vi "CPP-BLplotter.vi"(0 "Plot Array":cluster{dbl[], dbl[]}[](array[cluster])=[{[500.0, 500.0, 953.54, 215.0, 270.0, 320.0, 445.0, 525.0, 600.0, 675.0, 750.0, 825.0, 900.0, 960.0, 1010.0, 1060.0], [4.614524, 4.54365, 5.818368, 0.1374656, 0.6662545, 1.465458, 3.619824, 4.848976, 5.887329, 5.940571, 6.152151, 5.717487, 5.600293, 5.40069, 5.154843, 5.121789]}, {[100.0, 150.0, 215.0, 270.0, 320.0, 445.0, 525.0, 600.0, 675.0, 750.0, 825.0, 900.0, 960.0, 1010.0, 1060.0], [0.002314715, -0.00693192, 0.120417, 0.6880509, 1.519176, 3.513709, 5.065183, 6.116033, 6.096773, 5.938465, 5.593788, 5.5597, 5.387002, 5.304077, 4.887903]}] {"?" format="%.2f"; "?" format="%.2f"}, 1 "Job Directory":path=path "/G4_2_HD/Users/paulhayden/Documents/Projects/Westlakes_resolution") -> (2 "Saved Automatically?":bool, 3 "gnuplotScript":string="set term epslatex\nset output \"Plot.eps\"\nset xlabel '$Distance~(m)$'\nset ylabel '$DF~(s/m^3)\\times10^6$'\nset samples 1000\nset pointsize 1.00\nset title '$B38~Centreline~Glc$' 0, 0\nset size 0.75,0.9\n\n#set key 450, -2.5833\n unset key\nset label 1 '~~~~~~~~~~~Angle~(deg)~=~0' at -100, -2.58\nset label 2 '~~~~~~~~~~~Height~(m)~=~5' at -100, -3.27\n set xrange [0 : 500] \n# set autoscale x \n set yrange [0.10000 : 7]\n# set autoscale y \n\nplot \"B38_Centreline_Glc.dat\" index 0 using 1:2 axes x1y1 title '$File=B38R~DDD.xls$' with points 1 1, \\\n\"B38_Centreline_Glc.dat\" index 1 using 1:2 axes x1y1 title '$File=B38R~DDD~1.xls$' with points 1 3", 4 "Plot data file":path)   [LabVIEW 2013]
uses:
  Results_plotter_Global.vi
panel:
  in  "Tab Control":enum32{"Good Shit", "Boring Shit"}(tab)
  out "lambda-":dbl format="%_2g"
  out "lambda+":dbl format="%_2g"
  out "lambda(h)":dbl format="%.3g"
  in  "HeightJitter%":dbl=0.03 min=0.0 max=20.0 step=1.0
  in  "Spectra Folder::":path
  out "Spectrum":cluster{"all rows":dbl[], "all rows":dbl[]}[](graph)
  in  "Cancel Button":bool
  in  "Print Button":bool
  out "U,L(U)":cluster{dbl[], dbl[]}[](graph)
  out "TI,Sigma":cluster{dbl[], dbl[]}[](graph)
  in  "MaxFitFreq":dbl
  in  "U(h)":dbl
  in  "lambdaSpan(%)":dbl
  in  "integralTweak":dbl=1.0 min=0.8 max=1.2 step=0.01
  in  "Use for:":enum16{"\nU", "\nLambda", "\nTI", "\nSigma"}[](array[ring])=[enum."\nU", enum."\nTI", enum."\nSigma", enum."\nLambda"]
  out "Incoming Titles":string[](array[string])
  in  "Plot Title":u16(ring) items=["Title String Only", "Number of Measurements", "Date::", "Profile::", "Multi Run:Start Time:", "Multi Run:Row:Type", "Multi Run:Row:Number", "Point:Time:", "Time:Stamp:", "Measuring:Instrument:Type", "Comments::", "Run:Messages:", "X_{HF}:(mm):", "Y_{HF}:(mm):", "Z_{HF}:(mm):", "X_{5HP}:(mm):", "Y_{5HP}:(mm):", "Z_{5HP}:(mm):", "Repeat::", "U_{HF}/U_{ref}::", "TI_{HF}:%:", "\\sigma_{HF}/U_{ref}::", "L(U):Est:(m)", "U_{5HP}/U_{ref}::", "U_{HF}/U_{5HP}::", "TI_{U(5HP)}:%:", "Vmag_{5HP}/U_{ref}::", "V_{5HP}/U_{5HP}::", "W_{5HP}/U_{5HP}::", "U_{ref}::", "U_{HF}::", "Tau(HF)::", "uhf^2::", "uhf^3/(uhf^2)^1.5::", "(uhf^4/(uhf^2)^2) -3::", "HW (Uhf):Standard Error:in Mean", "HW (Uhf):Standard Error:in Variance", "HW:Cal:", "Vmag_{5HP}::", "U_{5HP}::", "V_{5HP}::", "W_{5HP}::", "Vmag_SD::", "U_SD::", "V_SD::", "W_SD::", "Tau(5HP1)::(nose)", "Tau(5HP2)::(bottom)", "Tau(5HP3)::(top)", "Tau(5HP4)::(side)", "Tau(5HP5)::(side)", "GoodFraction::", "5HP:Mode:", "5HP:ReturnType:", "Reference:Temperature:Used for Corrections", "Atmos:Pressure:Used for Corrections", "Av Analogue:Sampling:Rate", "No of:Analogue:Samples", "No Of:Measurement:Blocks", "Flow:Measurement:Time", "X:(URef):(mm)", "Y:(URef):(mm)", "Z:(URef):(mm)", "Original:Results:Filename", "Current:Data:Filename", "Current:Data File:1st Folder level", "Current:Data File:2nd Folder level", "Current:Data File:3rd Folder level", "Current:Data File:4th Folder level", "Current:File:Number", "Raw:Data:Filename"]
  in  "Filename Max length":i32=255
  out "Final Title":string="B38 Centreline Glc"
  out "Path":path
  in  "Plot Title Post Block":string
  in  "Plot Title Pre Block":string
  in  "Show Script Editor?":bool
  out "t":string
  in  "OpenLogfile?":bool
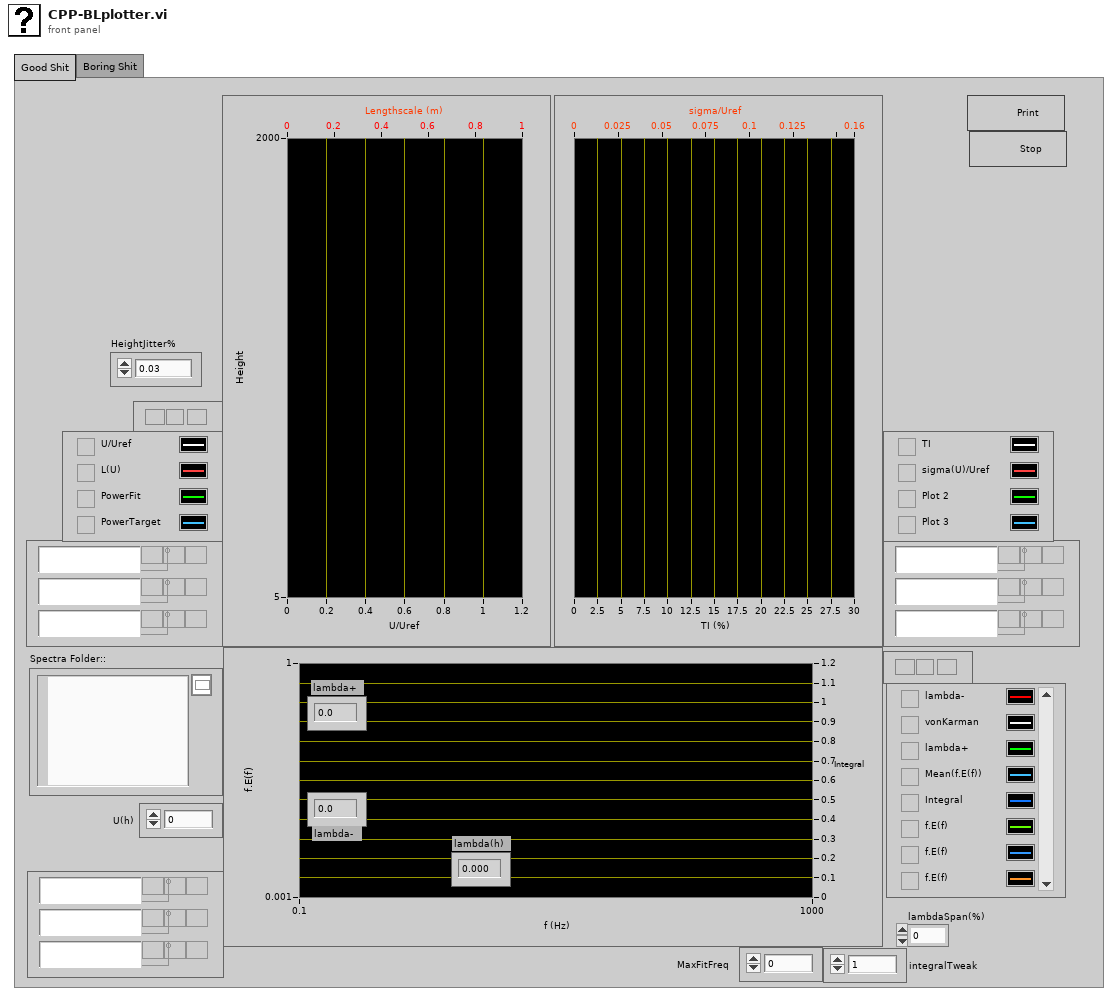
[diagram p1: front panel]
types:
  T1 = typedef "LVRangeTypeDef.ctl" = cluster{"Minimum":dbl, "Maximum":dbl, "Increment":dbl, "Minor Increment":dbl, "Start":dbl}
  T2 = cluster{"Array":dbl[], "best nonlinear fit":dbl[]}
  T3 = typedef "minAndMax.ctl" = cluster{"Min":T4, "Max":T4}
  T4 = typedef "AutoManualNumber.ctl" = cluster{"Auto":bool, "Value":dbl}
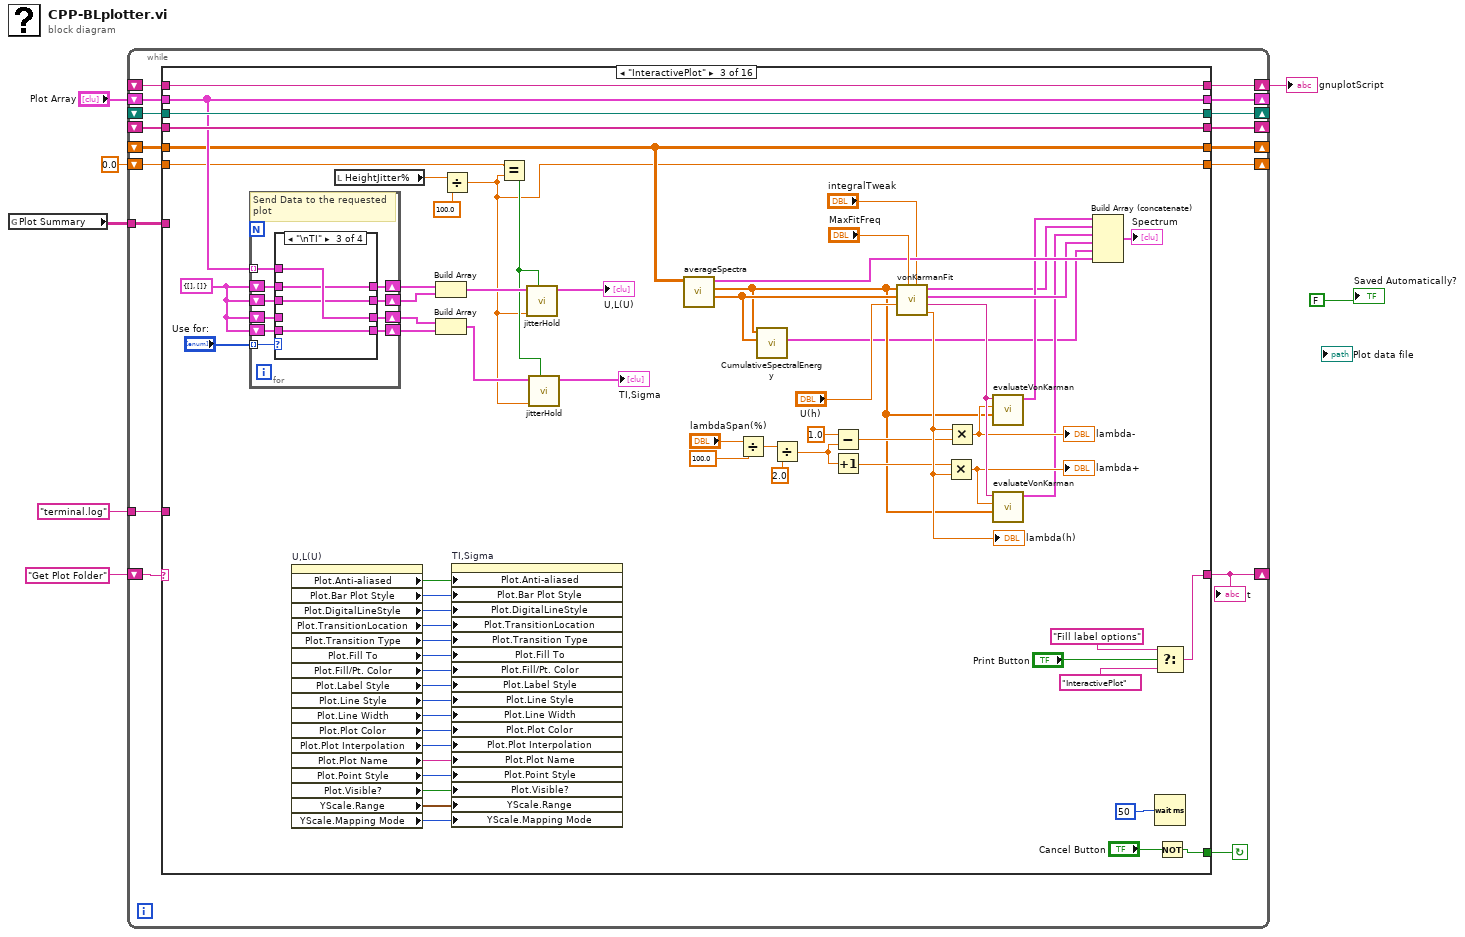
[diagram p0: block diagram]
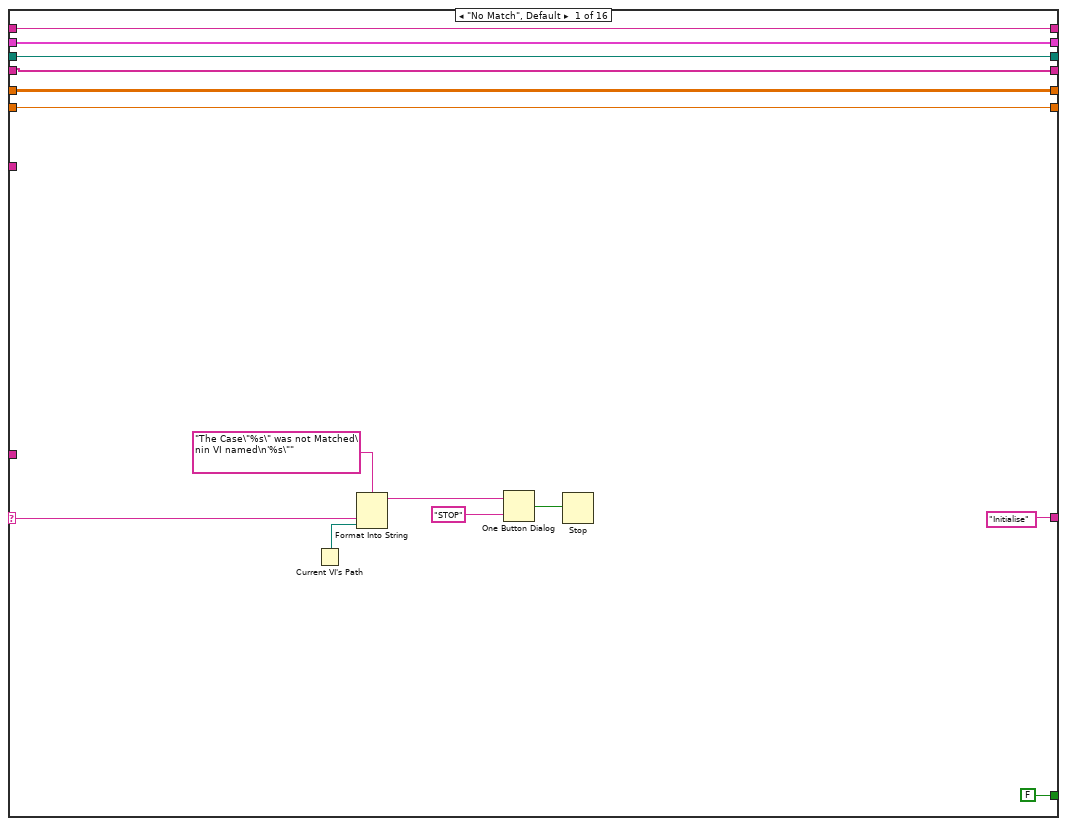
[diagram p2: hidden frame]
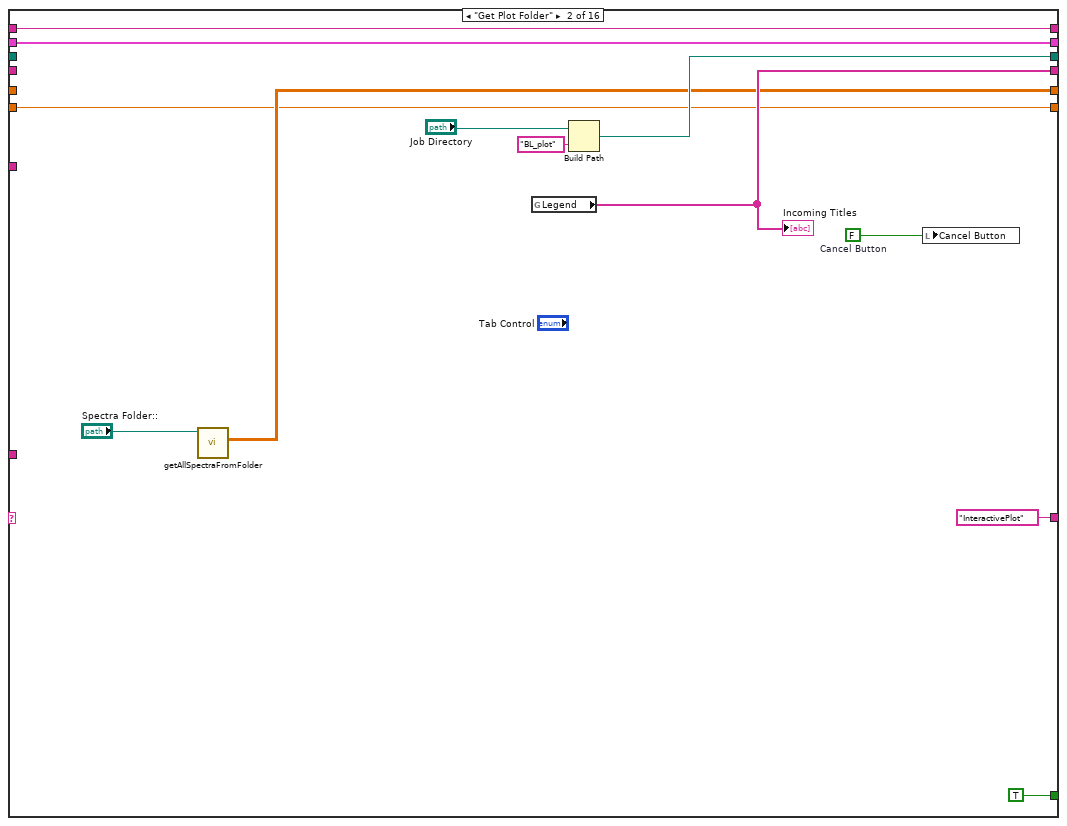
[diagram p3: hidden frame]
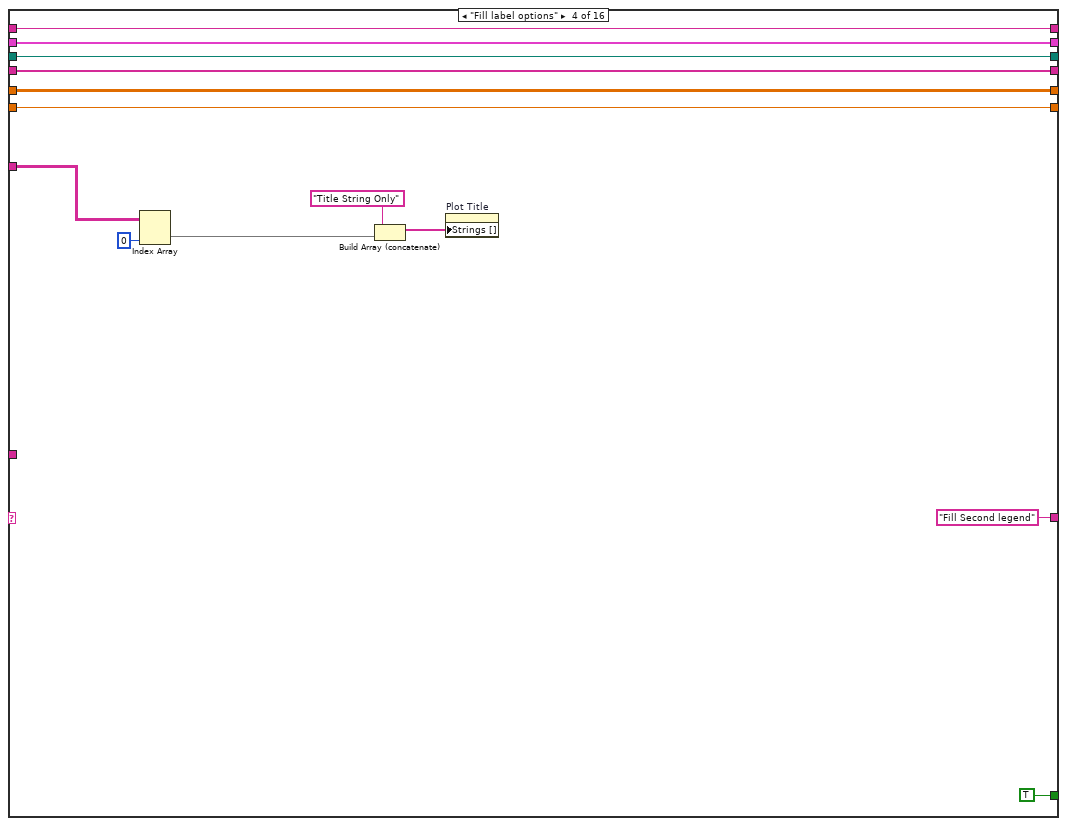
[diagram p7: hidden frame]
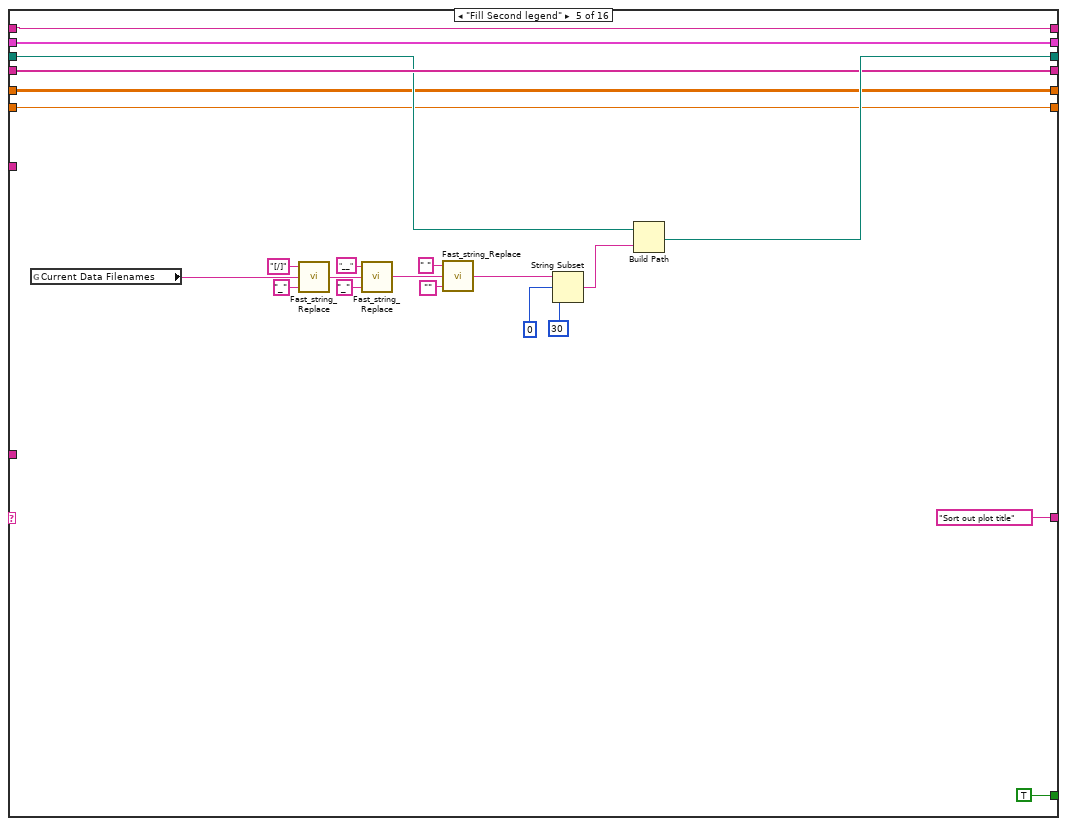
[diagram p8: hidden frame]
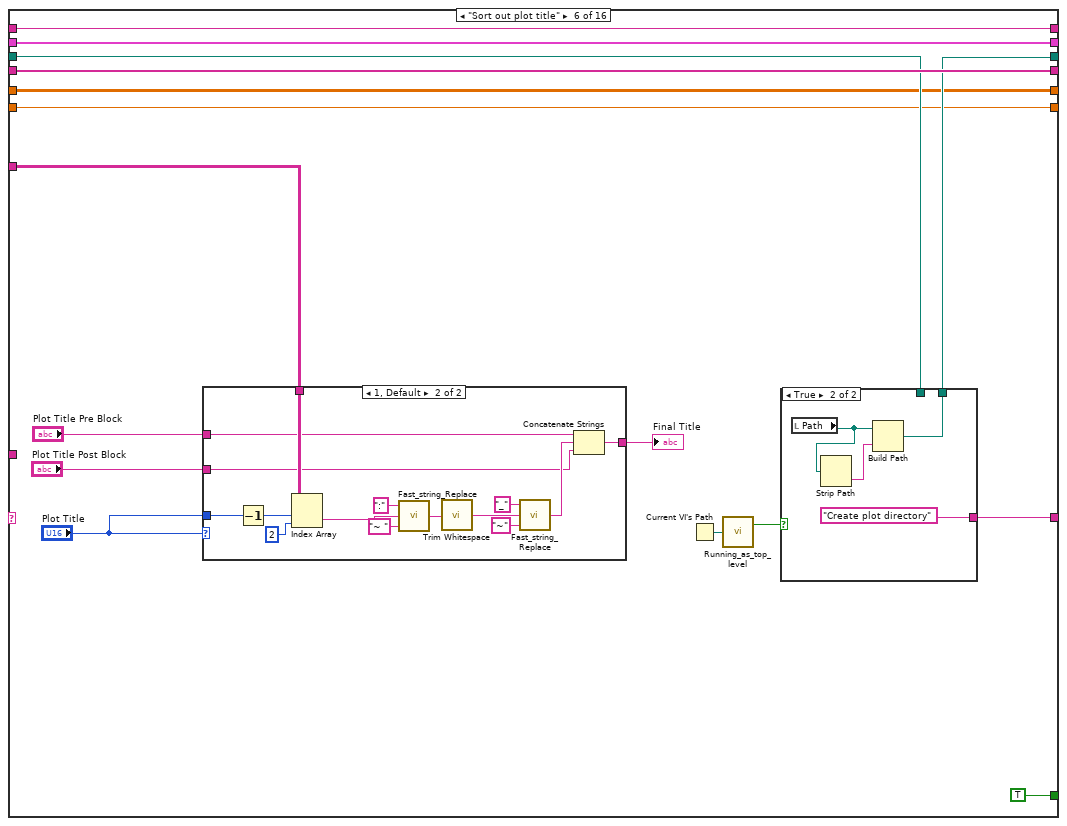
[diagram p9: hidden frame]
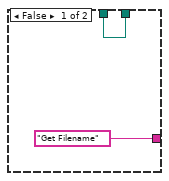
[diagram p10: hidden frame]
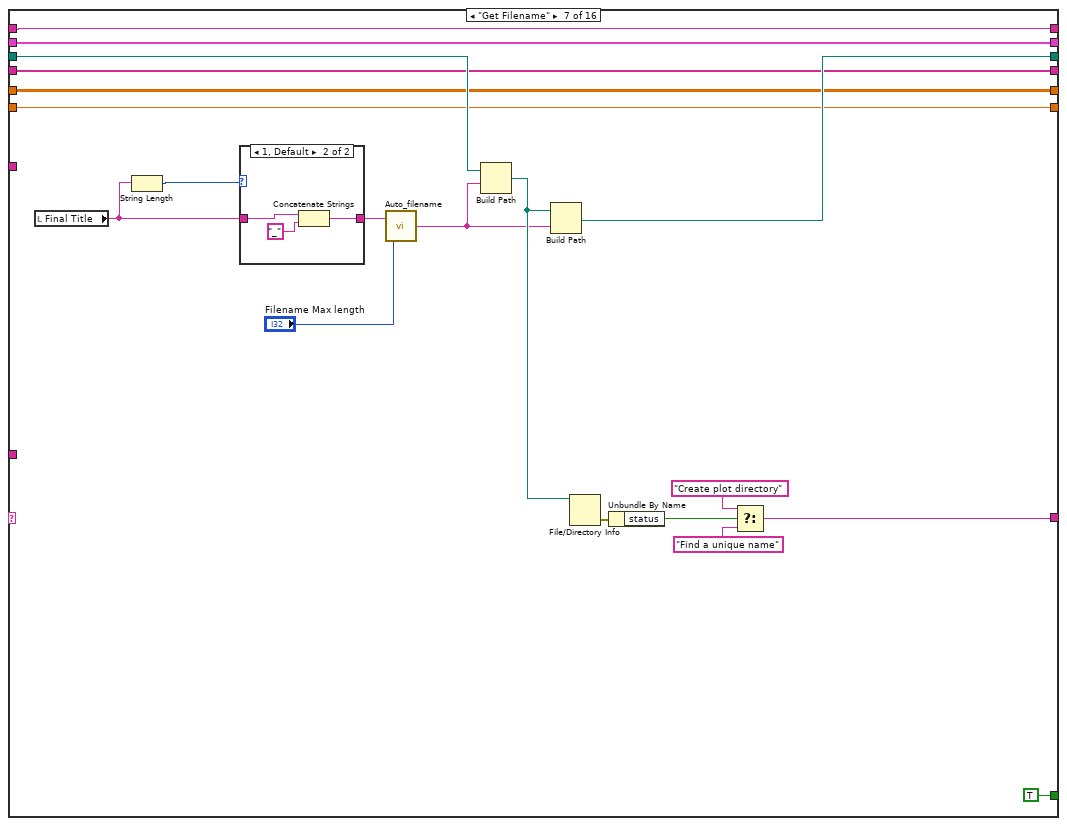
[diagram p12: hidden frame]
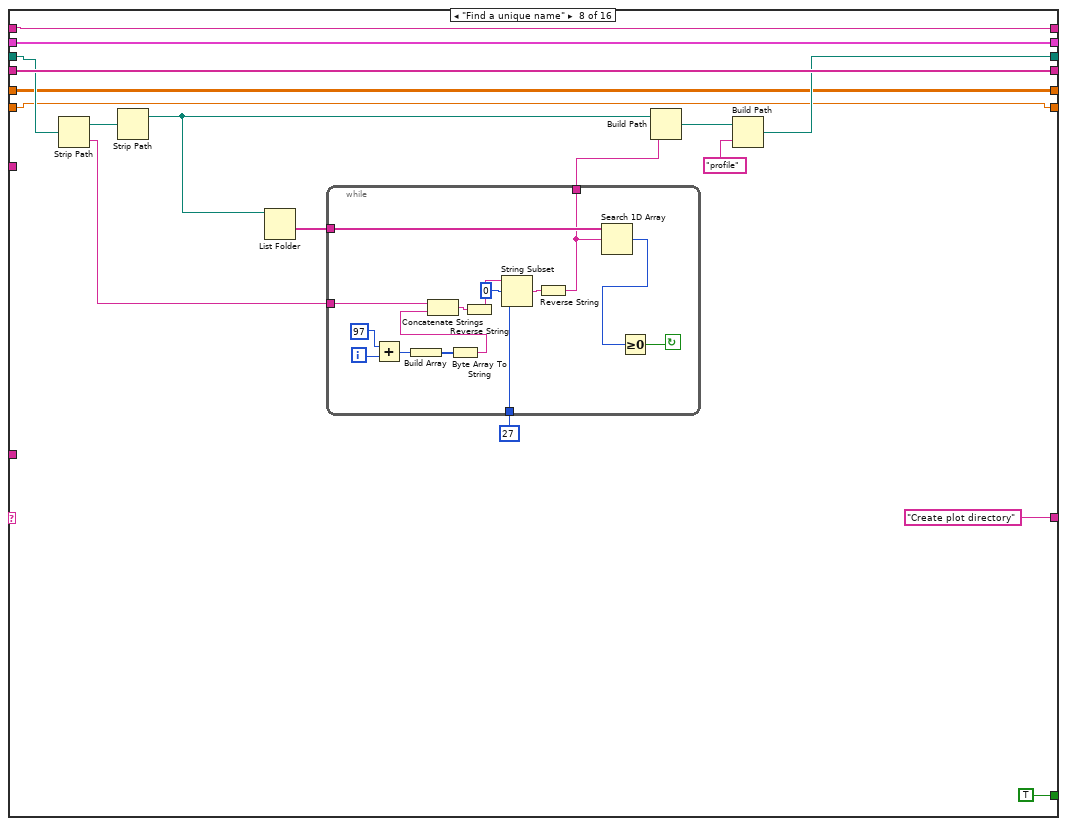
[diagram p14: hidden frame]
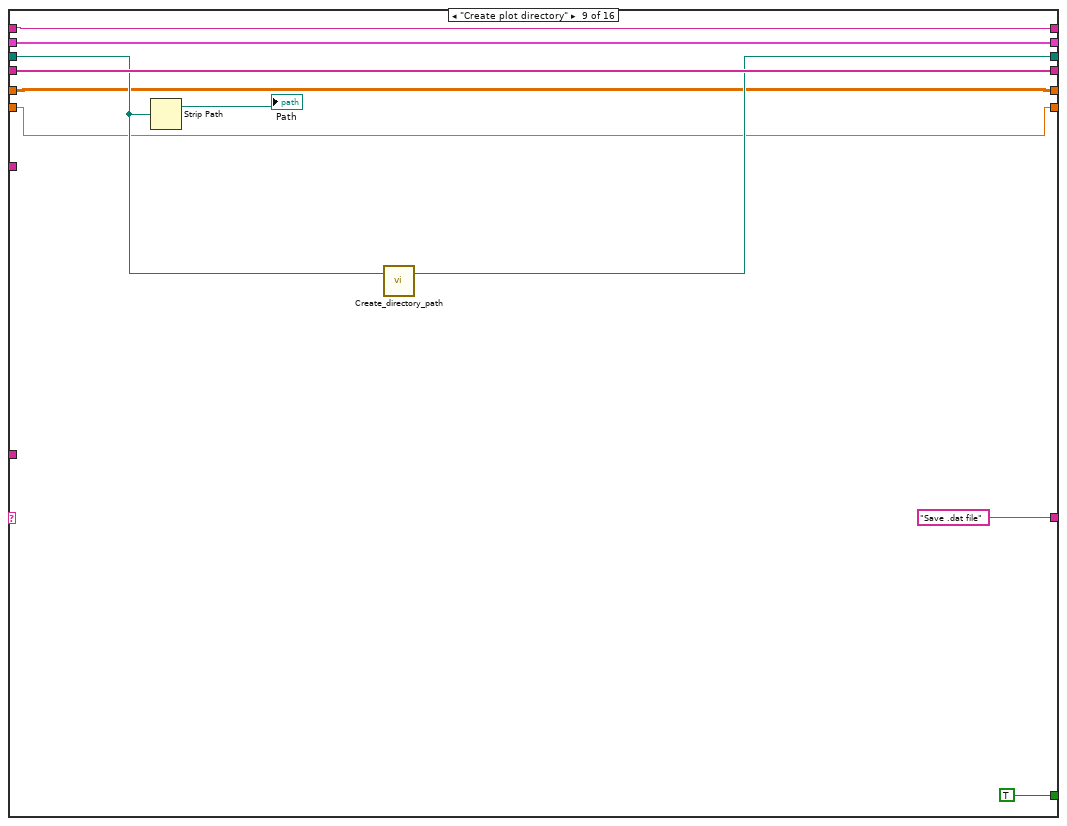
[diagram p15: hidden frame]
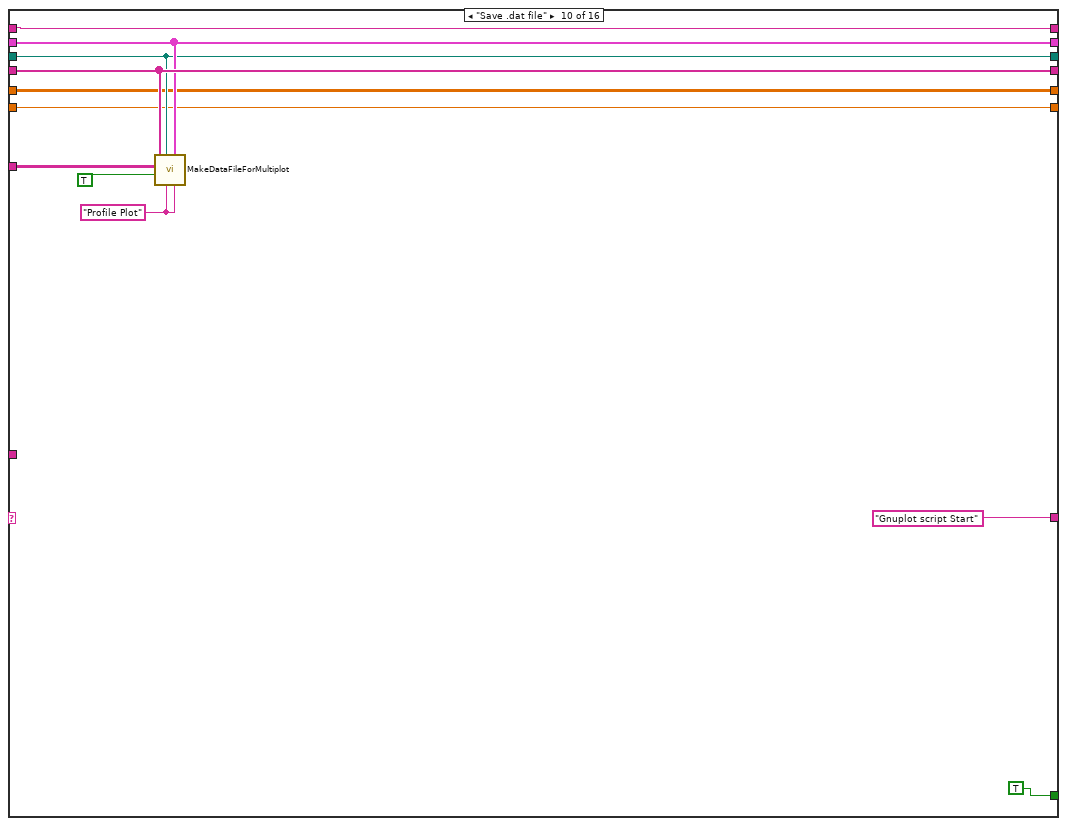
[diagram p16: hidden frame]
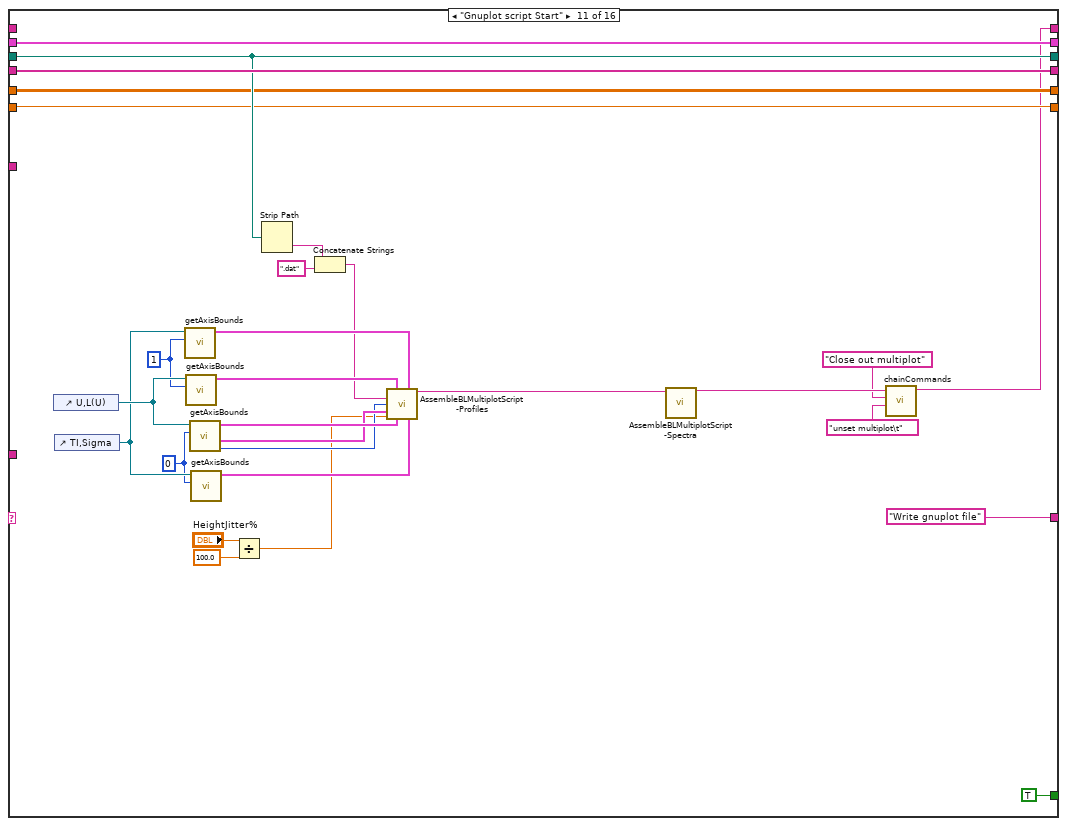
[diagram p17: hidden frame]
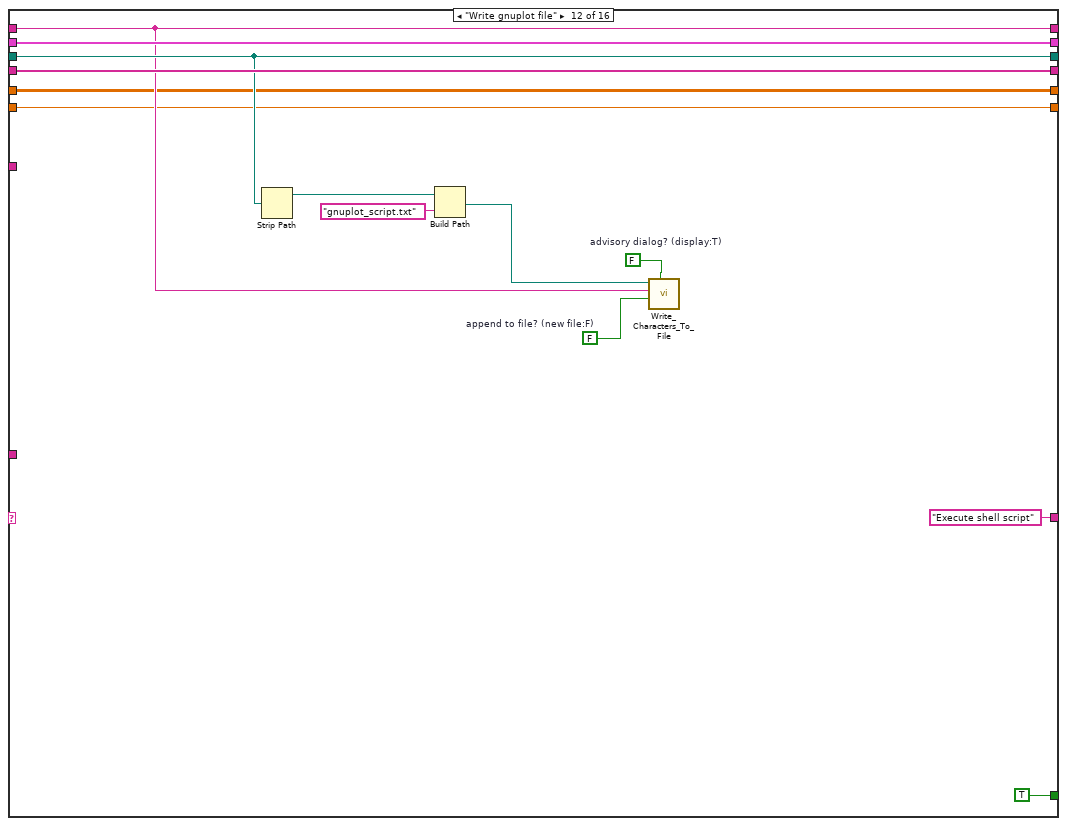
[diagram p18: hidden frame]
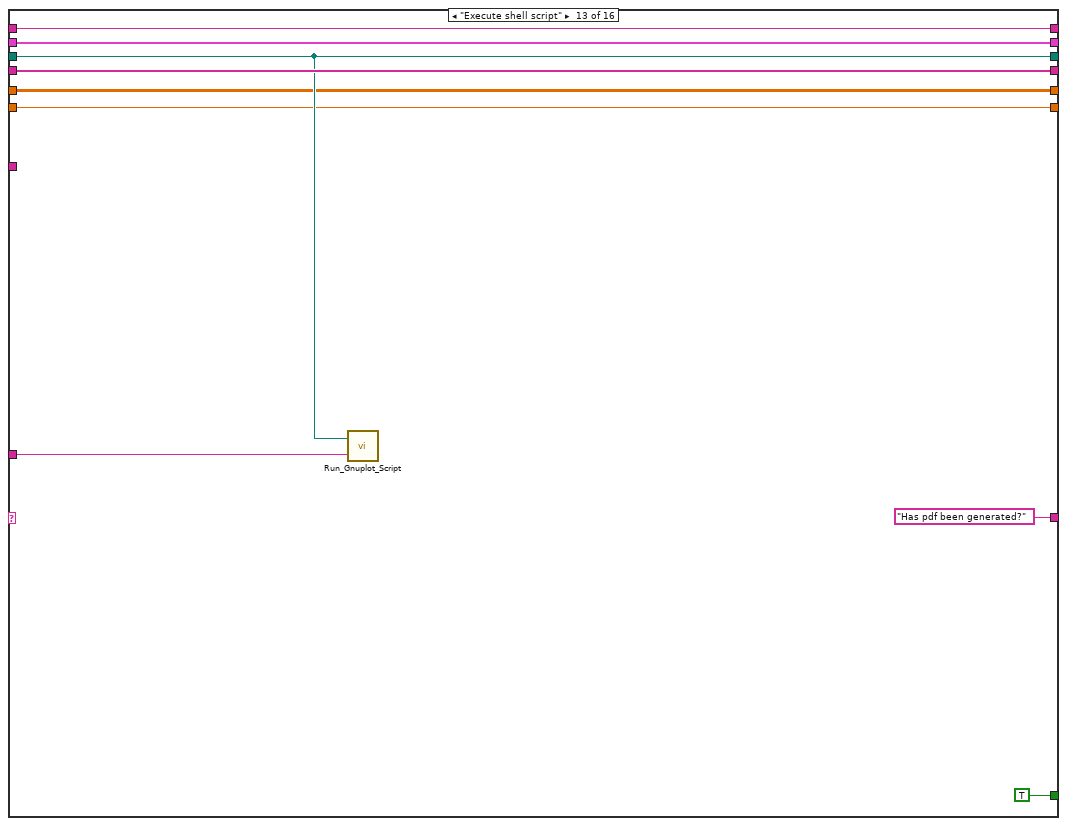
[diagram p19: hidden frame]
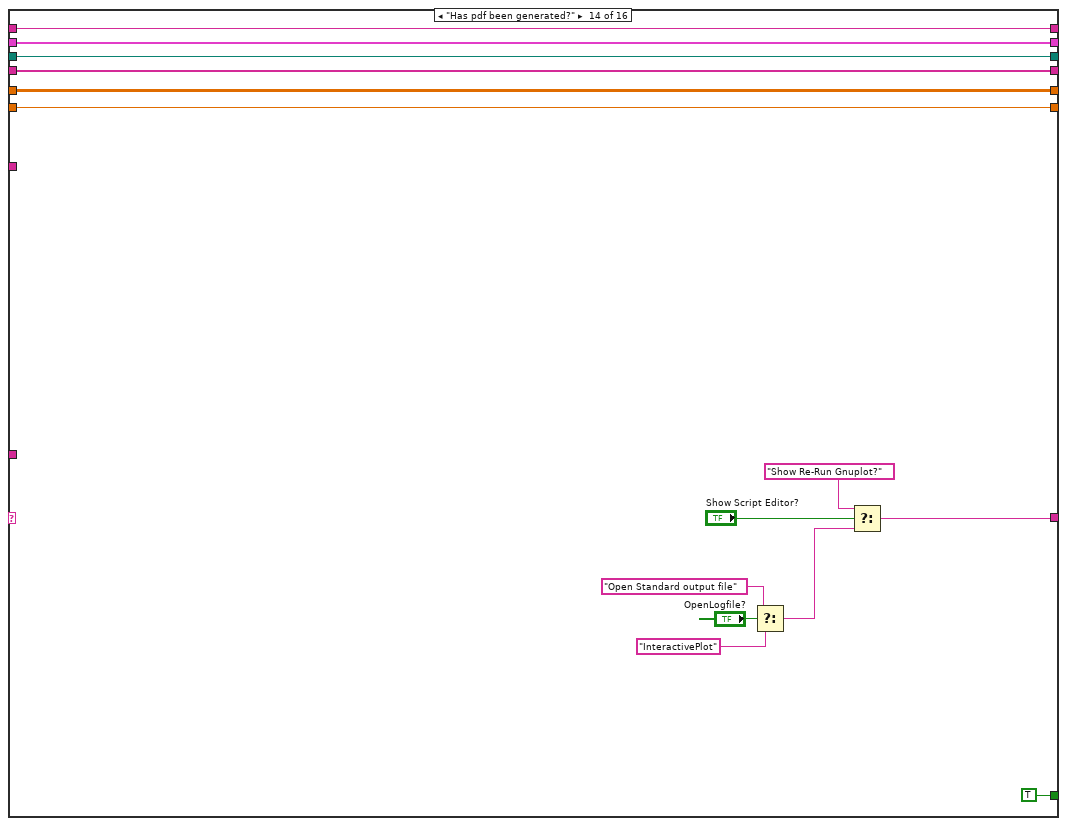
[diagram p20: hidden frame]
diagram:
  n1 = global read "Results_plotter_Global.vi" "Plot Summary"() -> (w6:string[][])
  n2 = while {
    shift-left: "Get Plot Folder" -> [w23]
    shift-right: [w12] -> _
    tunnel: w6 -> [w22]
    shift-right: [w21] -> _
    shift-left: _ -> [w20]
    shift-right: [w18] -> _
    shift-left: "Plot Array" -> [w19]
    shift-right: [w16] -> w5
    shift-left: _ -> [w17]
    shift-right: [w15] -> _
    shift-left: _ -> [w14]
    tunnel: "terminal.log" -> [w13]
    shift-right: [w11] -> _
    shift-left: _ -> [w10]
    shift-right: [w8] -> _
    shift-left: 0.0 ("HeightJitter%") -> [w9]
    stop <- w24 continue-if-true
    n3 = case shown="\"InteractivePlot\"" w23 {
      selector: w23 -> [w27 _ _ _ _ _ _ _ _ _ _ _ _ _ _ _]
      tunnel: [FALSE TRUE w110 TRUE ("Top Level") TRUE ("Top Level") TRUE ("Top Level") TRUE ("Top Level") TRUE ("Top Level") TRUE TRUE ("Top Level") TRUE ("Top Level") TRUE ("Top Level") TRUE ("Top Level") TRUE ("Top Level") TRUE ("Top Level") TRUE ("Top Level")] -> w24
      tunnel: ["Initialise" "InteractivePlot" w115 "Fill Second legend" "Sort out plot title" w183 w234 "Create plot directory" "Save .dat file" "Gnuplot script Start" "Write gnuplot file" ("t") "Execute shell script" ("t") "Has pdf been generated?" ("t") w350 "End" "InteractivePlot" ("t")] -> w12
      tunnel: w22 -> [_ _ _ w157 _ w190 _ _ _ w290 _ _ _ _ _ _]
      tunnel: [w31 w47 w118 w151 w179 w185 w235 w244 w279 w287 w318 w328 w338 w354 w361 w373] -> w21
      tunnel: w20 -> [w31 _ w118 w151 w175 w184 w231 w251 w278 w287 w318 w328 w338 w354 w361 w373]
      tunnel: w19 -> [w30 w44 w87 w152 w178 w195 w233 w254 w282 w288 w321 w334 w343 w357 w366 w378]
      tunnel: [w30 w44 w87 w152 w178 w195 w233 w254 w282 w288 w321 w334 w343 w357 w366 w378] -> w18
      tunnel: w17 -> [w29 w46 w116 w153 w177 w191 w232 w253 w281 w293 _ w324 w341 w355 w364 w376]
      tunnel: [w29 w46 w116 w153 w177 w191 w232 w253 w281 w293 w296 w324 w341 w355 w364 w376] -> w16
      tunnel: [w28 w42 w117 w150 w176 w194 w230 w252 w280 w289 w320 w329 w342 w356 w365 w377] -> w15
      tunnel: w14 -> [w28 _ w117 w150 w176 w194 w230 w252 w280 w289 w320 w329 w342 w356 w365 w377]
      tunnel: w13 -> [_ _ _ _ _ _ _ _ _ _ _ _ w337 _ _ w371]
      tunnel: [w26 w40 w79 w146 w159 w181 w219 w242 w274 w284 w301 w323 w336 w345 w359 w368] -> w11
      tunnel: w10 -> [w26 _ w79 w146 w159 w181 w219 w242 w274 w284 w301 w323 w336 w345 w359 w368]
      tunnel: w9 -> [w25 w39 w55 w145 w158 w180 w218 w241 w273 w283 w300 w322 w335 w344 w358 w367]
      tunnel: [w25 w39 w53 w145 w158 w180 w218 w241 w273 w283 w300 w322 w335 w344 w358 w367] -> w8
      frame "No Match", Default {
        n4 = Current VI's Path() -> (path=w33:path)
        n5 = Format Into String(format string="The Case\"%s\" was not Matched\nin VI named\n'%s\"" ("Format String"), w27, w33) -> (resulting string=w36:string)  [unwired: 2 in, 1 out]
        n6 = One Button Dialog(message=w36, button name ("OK")="STOP") -> (true=w34:bool)
        n7 = Stop(stop? (T)=w34) -> ()
      }
      frame "Get Plot Folder" {
        w43 = FALSE  # Cancel Button
        n8 = call "getAllSpectraFromFolder.vi"("Spectra Folder::"="Spectra Folder::") -> ("spectra"=w40:dbl[][][])  [unwired: 10 in]
        n9 = global read "Results_plotter_Global.vi" "Legend"() -> (w42:string[])
        "Incoming Titles" <- w42
        n10 = Build Path(base path="Job Directory", name or relative path="BL_plot") -> (appended path=w47:path)
        n11 = local write "Cancel Button"(w43) -> ()
      }
      frame "InteractivePlot" {
        w86 = cluster{dbl[], dbl[]} {[], []}
        n12 = for {
          tunnel: "Use for:" -> [w123] mode=indexing
          shift-right: [w128] -> w91
          shift-left: w86 -> [w122]
          shift-right: [w125] -> w89
          shift-left: w86 -> [w121]
          shift-right: [w124] -> w88
          shift-left: w86 -> [w120]
          shift-right: [w126] -> w90
          shift-left: w86 -> [w127]
          tunnel: w87 -> [w119] mode=indexing
          # "Send Data to the requested plot"
          n13 = case shown="\"\\nTI\"" w123 {
            tunnel: [w132 w134 w138 w143] -> w128
            tunnel: w127 -> [_ w133 w139 w144]
            tunnel: [w129 w133 w139 w144] -> w126
            tunnel: [w131 w136 w140 w142] -> w125
            tunnel: [w130 w135 w137 w141] -> w124
            tunnel: w122 -> [w132 _ w138 w143]
            tunnel: w121 -> [w131 w136 _ w142]
            tunnel: w120 -> [w130 w135 w137 _]
            tunnel: w119 -> [w129 w134 w140 w141]
            frame "\nU", Default {
            }
            frame "\nLambda" {
            }
            frame "\nTI" {
            }
            frame "\nSigma" {
            }
          }
        }
        n14 = property on="U,L(U)" class="XYGraph (strict)"() -> ("Plot.Anti-aliased"=w92:bool, "Plot.Bar Plot Style"=w93:u8, "Plot.DigitalLineStyle"=w94:u8, "Plot.TransitionLocation"=w95:u8, "Plot.Transition Type"=w96:u8, "Plot.Fill To"=w97:i16, "Plot.Fill/Pt. Color"=w98:u32, "Plot.Label Style"=w99:u8, "Plot.Line Style"=w100:u8, "Plot.Line Width"=w101:u8, "Plot.Plot Color"=w102:u32, "Plot.Plot Interpolation"=w103:u8, "Plot.Plot Name"=w104:string, "Plot.Point Style"=w105:u8, "Plot.Visible?"=w106:bool, "YScale.Range"=w107:T1, "YScale.Mapping Mode"=w108:u8)  [unwired: 2 in, 2 out]
        n15 = local read "HeightJitter%"() -> (w54:dbl)
        n16 = Build Array(w90, w91) -> (w58:cluster{dbl[], dbl[]}[])
        n17 = Build Array(w89, w88) -> (w60:cluster{dbl[], dbl[]}[])
        n18 = Divide(x=w54, y=100.0) -> (x/y=w53:dbl)
        n19 = property on="TI,Sigma" class="XYGraph (strict)"("Plot.Anti-aliased"=w92, "Plot.Bar Plot Style"=w93, "Plot.DigitalLineStyle"=w94, "Plot.TransitionLocation"=w95, "Plot.Transition Type"=w96, "Plot.Fill To"=w97, "Plot.Fill/Pt. Color"=w98, "Plot.Label Style"=w99, "Plot.Line Style"=w100, "Plot.Line Width"=w101, "Plot.Plot Color"=w102, "Plot.Plot Interpolation"=w103, "Plot.Plot Name"=w104, "Plot.Point Style"=w105, "Plot.Visible?"=w106, "YScale.Range"=w107, "YScale.Mapping Mode"=w108) -> ()  [unwired: 2 in, 2 out]
        n20 = Equal?(x=w55, y=w53) -> (x = y?=w56:bool)
        n21 = call "jitterHold.vi"("jitterChanged?"=w56, "Y-jitter"=w53, "Array"=w58) -> ("Array 2"=→"U,L(U)":cluster{"Array":dbl[], "Array":dbl[]}[])  [unwired: 8 in]
        n22 = call "jitterHold.vi"("jitterChanged?"=w56, "Y-jitter"=w53, "Array"=w60) -> ("Array 2"=→"TI,Sigma":cluster{"Array":dbl[], "Array":dbl[]}[])  [unwired: 8 in]
        n23 = call "averageSpectra.vi"("multipleSpectra"=w79) -> ("meanSpectrum"=w63:dbl[], "frequencies"=w62:dbl[], "spectraPlots"=w82:cluster{"Array":dbl[], "Array":dbl[]}[])  [unwired: 8 in]
        n24 = Divide(x="lambdaSpan(%)", y=100.0) -> (x/y=w72:dbl)
        n25 = call "CumulativeSpectralEnergy.vi"("f.E(f)"=w63, "f"=w62) -> ("plottableBundle"=w61:cluster{"X":dbl[], "Array":dbl[]})  [unwired: 8 in, 1 out]
        n26 = Divide(x=w72, y=2.0 ("x")) -> (x/y=w65:dbl)
        n27 = Subtract(x=1.0, y=w65) -> (x-y=w74:dbl)
        n28 = Increment(x=w65) -> (x+1=w73:dbl)
        n29 = call "vonKarmanFit.vi"("integralTweak"="integralTweak", "MaxFitFreq"="MaxFitFreq", "U(h)"="U(h)", "f.E(f)"=w63, "f"=w62) -> ("lambda"=w75:dbl, "vonKarmanFitEquation"=w78:string, "CroppedData"=w81:cluster{"X Out":dbl[], "Y Out":dbl[]}, "FitCurve"=w67:T2)  [unwired: 3 in]
        "lambda(h)" <- w75
        n30 = Multiply(x=w73, y=w75) -> (x*y=w68:dbl)
        "lambda+" <- w68
        n31 = Multiply(x=w75, y=w74) -> (x*y=w69:dbl)
        "lambda-" <- w69
        n32 = call "evaluateVonKarman.vi"("frequencies"=w62, "lambda"=w69, "vonKarmanFitEquation"=w78) -> ("Cluster"=w70:cluster{"frequencies":dbl[], "Y Values":dbl[]})  [unwired: 8 in]
        n33 = call "evaluateVonKarman.vi"("frequencies"=w62, "lambda"=w68, "vonKarmanFitEquation"=w78) -> ("Cluster"=w66:cluster{"frequencies":dbl[], "Y Values":dbl[]})  [unwired: 8 in]
        n34 = Build Array (concatenate)(w70, w67, w66, w81, w61, w82) -> (→"Spectrum":cluster{"Array":dbl[], "Array":dbl[]}[])
        n35 = Select(t="Fill label options", s="Print Button", f="InteractivePlot") -> (s? t:f=w115:string)
        n36 = Wait (ms)(milliseconds to wait=u32 50) -> ()  [unwired: 1 out]
        n37 = Not(x="Cancel Button") -> (.not. x?=w110:bool)
      }
      frame "Fill label options" {
        n38 = Index Array(array=w157, index (col)=0 ("disabled index (col)")) -> (element=w148:string[])  [unwired: 1 in]
        n39 = Build Array (concatenate)("Title String Only", w148) -> (w147:string[])
        n40 = property on="Plot Title" class="Ring (strict)"("Strings []"=w147) -> ()  [unwired: 2 in, 2 out]
      }
      frame "Fill Second legend" {
        n41 = global read "Results_plotter_Global.vi" "Current Data Filenames"() -> (w164:string)
        n42 = call "Fast_string_Replace.vi"("Replace match with:"="_", "Input String"=w164, "regular expression"="[/]") -> ("Output String"=w168:string)  [unwired: 2 out]
        n43 = call "Fast_string_Replace.vi"("Replace match with:"="_", "Input String"=w168, "regular expression"="__") -> ("Output String"=w165:string)  [unwired: 2 out]
        n44 = call "Fast_string_Replace.vi"("Replace match with:"="", "Input String"=w165, "regular expression"=" ") -> ("Output String"=w163:string)  [unwired: 2 out]
        n45 = String Subset(string=w163, offset (0)=0, length (rest)=30 ("length (rest)")) -> (substring=w162:string)
        n46 = Build Path(base path=w175, name or relative path=w162) -> (appended path=w179:path)
      }
      frame "Sort out plot title" {
        n47 = case shown="1, Default" "Plot Title" {
          tunnel: [w202 w207] -> w189
          tunnel: "Plot Title Pre Block" -> [w202 w206]
          tunnel: w190 -> [_ w210]
          tunnel: "Plot Title" -> [_ w209]
          tunnel: "Plot Title Post Block" -> [_ w203]
          frame 0 {
          }
          frame 1, Default {
            n48 = Decrement(x=w209) -> (x-1=w208:u16)
            n49 = Index Array(array=w210, index (row)=w208, index (col)=u16 2 ("y")) -> (element=w213:string)
            n50 = call "Fast_string_Replace.vi"("Replace match with:"="~ ", "Input String"=w213, "regular expression"=":") -> ("Output String"=w212:string)  [unwired: 2 out]
            n51 = call <vilib>:"Trim Whitespace.vi"("string"=w212) -> ("trimmed string"=w211:string)  [unwired: 1 in]
            n52 = call "Fast_string_Replace.vi"("Replace match with:"="~", "Input String"=w211, "regular expression"="_") -> ("Output String"=w205:string)  [unwired: 2 out]
            n53 = Concatenate Strings(w206, w205, w203) -> (w207:string)
          }
        }
        "Final Title" <- w189
        n54 = Current VI's Path() -> (path=w188:path)
        n55 = call "Running_as_top_level.vi"("Vi path name"=w188) -> ("Top Level"=w186:bool)  [unwired: 1 out]
        n56 = case shown="True" w186 {
          tunnel: [w197 w200] -> w185
          tunnel: w184 -> [w197 _]
          tunnel: ["Get Filename" ("t") "Create plot directory"] -> w183
          frame False {
          }
          frame True {
            n57 = local read "Path"() -> (w199:path)
            n58 = Strip Path(path=w199) -> (name=w198:string)  [unwired: 1 out]
            n59 = Build Path(base path=w199, name or relative path=w198) -> (appended path=w200:path)
          }
        }
      }
      frame "Get Filename" {
        n60 = local read "Final Title"() -> (w220:string)
        n61 = String Length(string=w220) -> (length=w222:i32)
        n62 = case shown="1, Default" w222 {
          tunnel: [w237 w238] -> w221
          tunnel: w220 -> [w237 w240]
          frame 0 {
          }
          frame 1, Default {
            n63 = Concatenate Strings(w240, "_") -> (w238:string)
          }
        }
        n64 = call "Auto_filename.vi"("Filename Max length"="Filename Max length", "Prefix"=w221) -> ("Filename"=w224:string)
        n65 = Build Path(base path=w231, name or relative path=w224) -> (appended path=w228:path)
        n66 = Build Path(base path=w228, name or relative path=w224) -> (appended path=w235:path)
        n67 = File/Directory Info(path=w228) -> (error out=w229:errorcluster)  [unwired: 1 in, 6 out]
        n68 = Unbundle By Name(w229) -> ("status"=w227:bool)
        n69 = Select(t="Create plot directory", s=w227, f="Find a unique name") -> (s? t:f=w234:string)
      }
      frame "Find a unique name" {
        n70 = Strip Path(path=w251) -> (stripped path=w250:path, name=w249:string)
        n71 = Strip Path(path=w250) -> (stripped path=w247:path)  [unwired: 1 out]
        n72 = List Folder(path=w247) -> (folder names=w248:string[])  [unwired: 1 in, 5 out]
        n73 = while {
          tunnel: w249 -> [w272]
          tunnel: 27 ("Max Length") -> [w271]
          tunnel: [w260] -> w246
          tunnel: w248 -> [w261]
          i -> [w262]
          stop <- w258 continue-if-true
          n74 = Add(x=97, y=w262) -> (x+y=w269:i32)
          n75 = Build Array(w269) -> (w270:i32[])
          n76 = Byte Array To String(unsigned byte array=w270) -> (string=w267:string)
          n77 = Concatenate Strings(w272, w267) -> (w265:string)
          n78 = Reverse String(1:w265) -> (0:w266:string)
          n79 = String Subset(string=w266, offset (0)=0, length (rest)=w271) -> (substring=w264:string)
          n80 = Reverse String(1:w264) -> (0:w260:string)
          n81 = Search 1D Array(1D array=w261, element=w260) -> (index of element=w259:i32)  [unwired: 1 out]
          n82 = Greater Or Equal To 0?(x=w259) -> (x >= 0?=w258:bool)
        }
        n83 = Build Path(base path=w247, name or relative path=w246) -> (appended path=w245:path)
        n84 = Build Path(base path=w245, name or relative path="profile") -> (appended path=w244:path)
      }
      frame "Create plot directory" {
        n85 = Strip Path(path=w278) -> (stripped path=→"Path":path)  [unwired: 1 out]
        n86 = call "Create_directory_path.vi"("Path name"=w278) -> ("Path name Out"=w279:path)  [unwired: 1 in, 1 out]
      }
      frame "Save .dat file" {
        w285 = "Profile Plot" ("X Axis Name")
        n87 = call "MakeDataFileForMultiplot.vi"("Y Axis Name"=w285, "Plot Array"=w288, "X Axis Name"=w285, "Path"=w287, "Transpose"=TRUE, "Plot Summary"=w290, "Legend"=w289) -> ()  [unwired: 5 in]
      }
      frame "Gnuplot script Start" {
        w311 = 1 ("Active X Scale")
        w312 = 0 ("Active X Scale")
        n88 = control-ref of="U,L(U)"() -> (w314:refnum<vi>)
        n89 = control-ref of="TI,Sigma"() -> (w313:refnum<vi>)
        n90 = call "getAxisBounds.vi"("Active X Scale"=w311, "XYGraph in"=w313) -> ("Xbounds"=w310:T3)  [unwired: 6 in, 3 out]
        n91 = call "getAxisBounds.vi"("Active X Scale"=w311, "XYGraph in"=w314) -> ("Xbounds"=w309:T3)  [unwired: 6 in, 3 out]
        n92 = call "getAxisBounds.vi"("Active X Scale"=w312, "XYGraph in"=w314) -> ("YMapping"=w305:enum8{"Lin", "Log"}, "Ybounds"=w306:T3, "Xbounds"=w308:T3)  [unwired: 6 in, 1 out]
        n93 = call "getAxisBounds.vi"("Active X Scale"=w312, "XYGraph in"=w313) -> ("Xbounds"=w307:T3)  [unwired: 6 in, 3 out]
        n94 = Divide(x="HeightJitter%", y=100.0) -> (x/y=w304:dbl)
        n95 = Strip Path(path=w318) -> (name=w316:string)  [unwired: 1 out]
        n96 = Concatenate Strings(w316, ".dat" ("string")) -> (w299:string)
        n97 = call "AssembleBLMultiplotScript-Profiles.vi"("lambdaBounds"=w309, "sigma/U bounds"=w310, "ProfileFilename"=w299, "Mapping"=w305, "HeightAxisBounds"=w306, "jitterFraction"=w304, "U/UrefBounds"=w308, "TI bounds"=w307) -> ("gnuplotOut"=w298:string)  [unwired: 7 in]
        n98 = call "AssembleBLMultiplotScript-Spectra.vi"("gnuplotIn"=w298) -> ("gnuplotOut"=w297:string)  [unwired: 14 in]
        n99 = call "chainCommands.vi"("Command"="unset multiplot\t", "Comments"="Close out multiplot", "StringIn"=w297) -> ("StringOut"=w296:string)  [unwired: 8 in]
      }
      frame "Write gnuplot file" {
        w331 = FALSE  # append to file? (new file:F)
        w332 = FALSE  # advisory dialog? (display:T)
        n100 = Strip Path(path=w328) -> (stripped path=w325:path)  [unwired: 1 out]
        n101 = Build Path(base path=w325, name or relative path="gnuplot_script.txt") -> (appended path=w333:path)
        n102 = call "Write_Characters_To_File.vi"("file path (dialog if empty)"=w333, "advisory dialog? (display:T)"=w332, "character string"=w324, "append to file? (new file:F)"=w331) -> ()  [unwired: 1 in, 4 out]
      }
      frame "Execute shell script" {
        n103 = call "Run_Gnuplot_Script.vi"("logfileName"=w337, "workingDirectory"=w338) -> ()
      }
      frame "Has pdf been generated?" {
        n104 = Select(t="Open Standard output file" ("f"), s="OpenLogfile?", f="InteractivePlot" ("t")) -> (s? t:f=w347:string)
        n105 = Select(t="Show Re-Run Gnuplot?", s="Show Script Editor?", f=w347) -> (s? t:f=w350:string)
      }
      frame "Show Re-Run Gnuplot?" {
        (unwired) "InteractivePlot" ("t")
        n106 = Strip Path(path=w361) -> (stripped path=w360:path)  [unwired: 1 out]
        n107 = call "Re_run_Gnuplot.vi"("Plot folder (dialog if empty)"=w360) -> ()  [unwired: 4 out]
      }
      frame "Open Standard output file" {
        n108 = Strip Path(path=w373) -> (stripped path=w370:path)  [unwired: 1 out]
        n109 = Format Into String(format string="open \"%s\"", w371) -> (resulting string=w369:string)  [unwired: 2 in, 1 out]
        n110 = call <vilib>:"System Exec.vi"("working directory"=w370, "command line"=w369) -> ()  [unwired: 4 in, 6 out]
      }
    }
    "t" <- w12
  }
  "gnuplotScript" <- w5
  "Saved Automatically?" <- FALSE
